vi "SR201_set_state.vi"(8 "error in":errorcluster, 9 "state":bool, 10 "channel":enum16{"CH1", "CH2"}(ring), 11 "conn_id_in":refnum<k5>) -> (0 "error out":errorcluster, 1 "ch2":bool, 2 "ch1":bool, 3 "conn_id_out":refnum<k5>, 4 "status":bool, 5 "string":string)   [LabVIEW 2019]
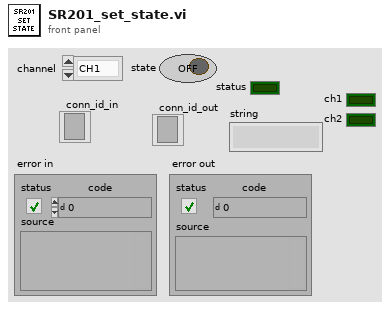
[diagram p1: front panel]
types:
  T1 = enum16{"Standard", "Buffered", "CRLF", "Immediate"}
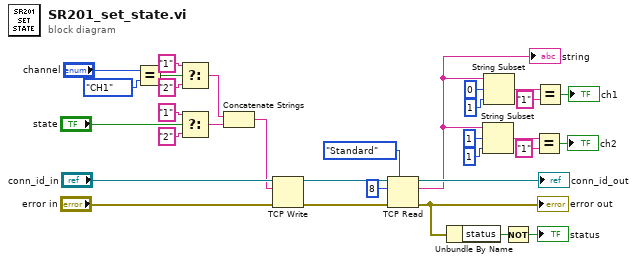
[diagram p0: block diagram]
diagram:
  n1 = Equal?(x="channel", y=enum16{"CH1", "CH2"}."CH1") -> (x = y?=w9:bool)
  n2 = Select(t="1", s=w9, f="2") -> (s? t:f=w3:string)
  n3 = Select(t="1", s="state", f="2") -> (s? t:f=w2:string)
  n4 = Concatenate Strings(w3, w2) -> (w1:string)
  n5 = TCP Write(connection ID="conn_id_in", data in=w1, error in (no error)="error in") -> (connection ID out=w30:refnum<k5>, error out=w31:errorcluster)  [unwired: 1 in, 1 out]
  n6 = TCP Read(connection ID=w30, bytes to read=8, error in (no error)=w31, 7:T1."Standard" ("mode (standard)")) -> (connection ID out=→"conn_id_out":refnum<k5>, data out=w12:string, error out=w25:errorcluster)  [unwired: 1 in]
  "error out" <- w25
  "string" <- w12
  n7 = Unbundle By Name(w25) -> ("status"=w24:bool)
  n8 = String Subset(string=w12, offset (0)=1, length (rest)=1 ("length (rest)")) -> (substring=w15:string)
  n9 = String Subset(string=w12, offset (0)=0, length (rest)=1 ("length (rest)")) -> (substring=w20:string)
  n10 = Not(x=w24) -> (.not. x?=→"status":bool)
  n11 = Equal?(x=w15, y="1") -> (x = y?=→"ch2":bool)
  n12 = Equal?(x=w20, y="1") -> (x = y?=→"ch1":bool)
